vi "Save Report to File.vi"(0 "report in":refnum<class "ooWriter.lvclass">, 5 "report file path":path, 7 "prompt to replace? (F)":bool, 9 "password (\"\")":string, 11 "error in (no error)":errorcluster) -> (4 "report out":refnum<class "ooWriter.lvclass">, 15 "error out":errorcluster)   [LabVIEW 2009, in "ooWriter.lvclass"]
doc: "Saves an HTML report to the file specified in <B>report file path</B>. You cannot use this VI with standard reports.\n\nThis VI also saves Microsoft Word and Excel reports."
uses:
  ooWriter.lvclass
  ooWriter.lvclass/ooWriter.ctl
  C:/Projets/LAVAG/OpenOfficeRGT/AODL/DLLs/AODL.dll
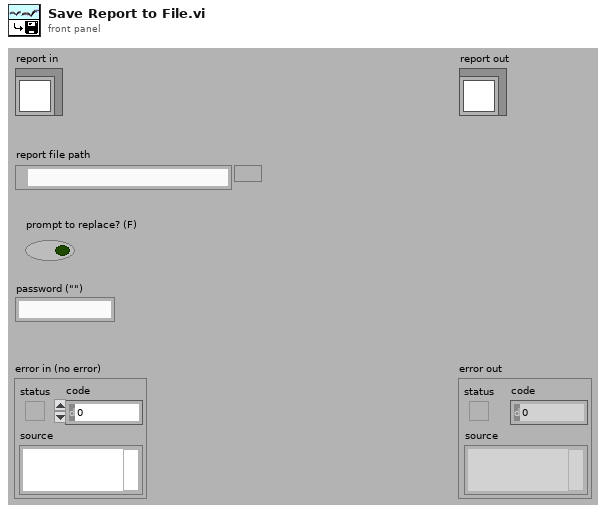
[diagram p1: front panel]
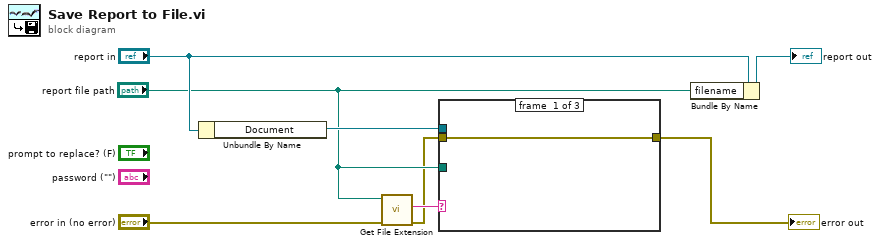
[diagram p0: block diagram]
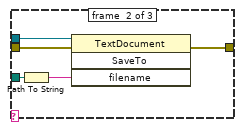
[diagram p2: hidden frame]
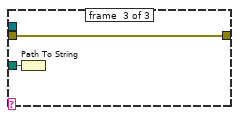
[diagram p3: hidden frame]
diagram:
  n1 = Unbundle By Name("report in") -> ("Document"=w5:refnum<k24>)
  n2 = call <vilib>:"Get File Extension.vi"("error in (no error)"="error in (no error)", "file"="report file path") -> ("error out"=w1:errorcluster, "lowercase file extension"=w4:string)  [unwired: 6 in, 2 out]
  n3 = case shown="\"odt\"" w4 {
    tunnel: w1 -> [w9 w14 w15]
    tunnel: w5 -> [_ w13 _]
    tunnel: [w9 w11 w15] -> w6
    tunnel: "report file path" -> [_ w10 w16]
    frame #0 {
    }
    frame #1 {
      n4 = Path To String(path=w10) -> (string=w12:string)
      n5 = invoke class="TextDocument" method="SaveTo"(reference=w13, error in=w14, "filename"=w12) -> (error out=w11:errorcluster)  [unwired: 1 in, 3 out]
    }
    frame #2 {
      n6 = Path To String(path=w16) -> ()  [unwired: 1 out]
    }
  }
  "error out" <- w6
  n7 = Bundle By Name(cluster="report in", "filename"="report file path") -> (→"report out":refnum<class "ooWriter.lvclass">)
